vi "Read Title Bar.vi"(11 "Flex Dialog in":refnum<class "Flex UI Dialog.lvclass">) -> (2 "Title Bar":bool, 3 "Flex Dialog out":refnum<class "Flex UI Dialog.lvclass">)   [LabVIEW 2016, in "Flex UI Dialog.lvclass"]
uses:
  Flex UI Dialog.lvclass
  Flex UI Dialog.lvclass/Flex UI Dialog.ctl
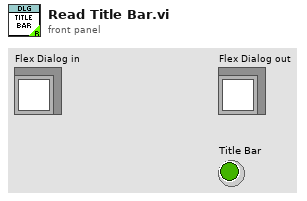
[diagram p1: front panel]
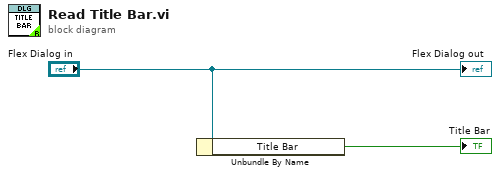
[diagram p0: block diagram]
diagram:
  n1 = Unbundle By Name("Flex Dialog in") -> ("Title Bar"=→"Title Bar":bool)
  "Flex Dialog out" <- "Flex Dialog in"
